vi "PathPlanner_EventMarker_SetMarkerPos.vi"(9 "MarkerPos":T1 {"Y" format="%14.3f"; "X" format="%14.3f"}, 11 "in EventMarker":T2 {"lastRobotPos"."Y" format="%14.3f"; "lastRobotPos"."X" format="%14.3f"; "markerPos"."Y" format="%14.3f"; "markerPos"."X" format="%14.3f"}) -> (3 "out EventMarker":T2 {"lastRobotPos"."Y" format="%14.3f"; "lastRobotPos"."X" format="%14.3f"; "markerPos"."Y" format="%14.3f"; "markerPos"."X" format="%14.3f"})   [LabVIEW 2019, in "PathPlanner24.lvlib"]
doc: "Get the marker position for this event\n \nInputs:\n - EventMarker - cluster - Data cluster\n - MarkerPos - double - Marker position\n\nOutputs:\n - EventMarker - cluster - Data cluster"
uses:
  PathPlanner24.lvlib
  TypeDef/PathPlannerEventMarker.ctl
  <vilib>/Rock Robotics/WPI/ThirdParty/JAS_Junk/TrajLib/TypeDef/TRANSLATION2D.ctl
  TypeDef/PathPlannerCommandUtil.ctl
  ENum/PathPlanner_CommandUtilType_ENUM.ctl
  <vilib>/Rock Robotics/WPI/ThirdParty/JAS_Junk/TrajLib/Trajectory_Library.lvlib
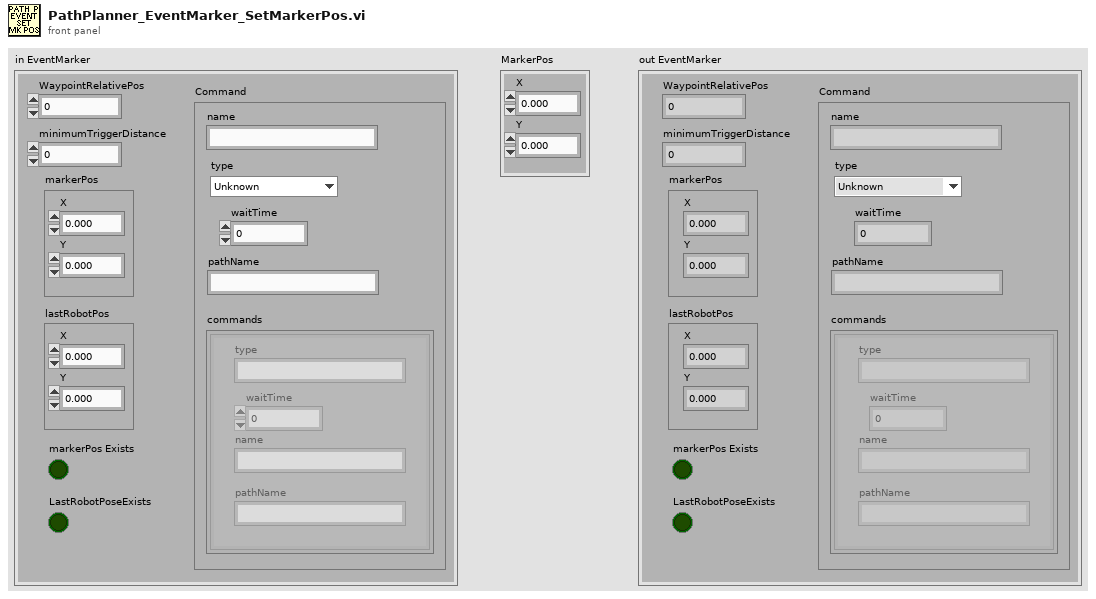
[diagram p1: front panel]
types:
  T1 = typedef "Trajectory_Library.lvlib/TRANSLATION2D.ctl" = cluster{"X":dbl, "Y":dbl}
  T2 = typedef "PathPlanner24.lvlib/PathPlannerEventMarker.ctl" = cluster{"WaypointRelativePos":dbl, "minimumTriggerDistance":dbl, "markerPos":T1, "lastRobotPos":T1, "Command":T3, "markerPos Exists":bool, "LastRobotPoseExists":bool}
  T3 = typedef "PathPlanner24.lvlib/PathPlannerCommandUtil.ctl" = cluster{"waitTime":dbl, "name":string, "pathName":string, "commands":cluster{"type":string, "waitTime":dbl, "name":string, "pathName":string}[], "type":T4}
  T4 = typedef "PathPlanner24.lvlib/PathPlanner_CommandUtilType_ENUM.ctl" = enum16{"Unknown", "Wait", "Named", "Path", "Sequential", "Parallel", "Race", "Deadline"}
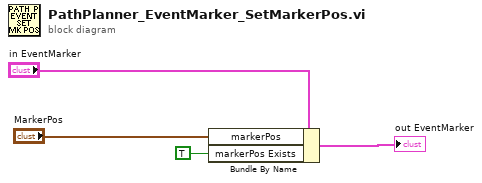
[diagram p0: block diagram]
diagram:
  n1 = Bundle By Name(cluster="in EventMarker", "markerPos"="MarkerPos", "markerPos Exists"=TRUE ("LastRobotPoseExists")) -> (→"out EventMarker":T2)
